vi "Open DQMH MHL Request Case QD.vi"(6 "Variant in":variant, 7 "Shift Pressed?":bool, 8 "error in (no error)":errorcluster, 10 "QD Combo Box Ref":refnum<vi>, 11 "QD Launch VI Ref":refnum<vi>) -> (0 "error out":errorcluster, 4 "Variant out":variant)   [LabVIEW 2017]
doc: "Write a 1-2 sentence description of the functionality of your plugin here. Replace the \"$\" below with the character you wish to assign as the default shortcut for this plugin. Do not add any text after the 'Default Shortcut' line below.\n\nDefault Shortcut - [k]"
panel:
  in  "Undo Name":string="Quick Drop Keyboard Shortcut"
  # "Do not change the connector pane of this VI.\n\nSee the block diagram for directions on how to use this template."
  # "Specify the name of the Undo transaction"
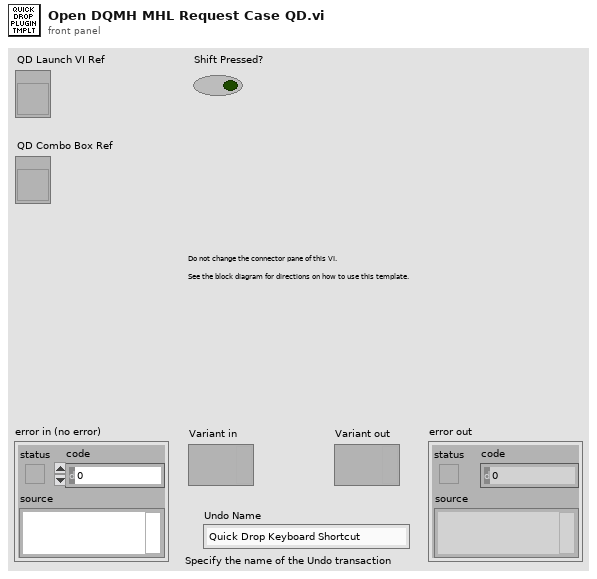
[diagram p1: front panel]
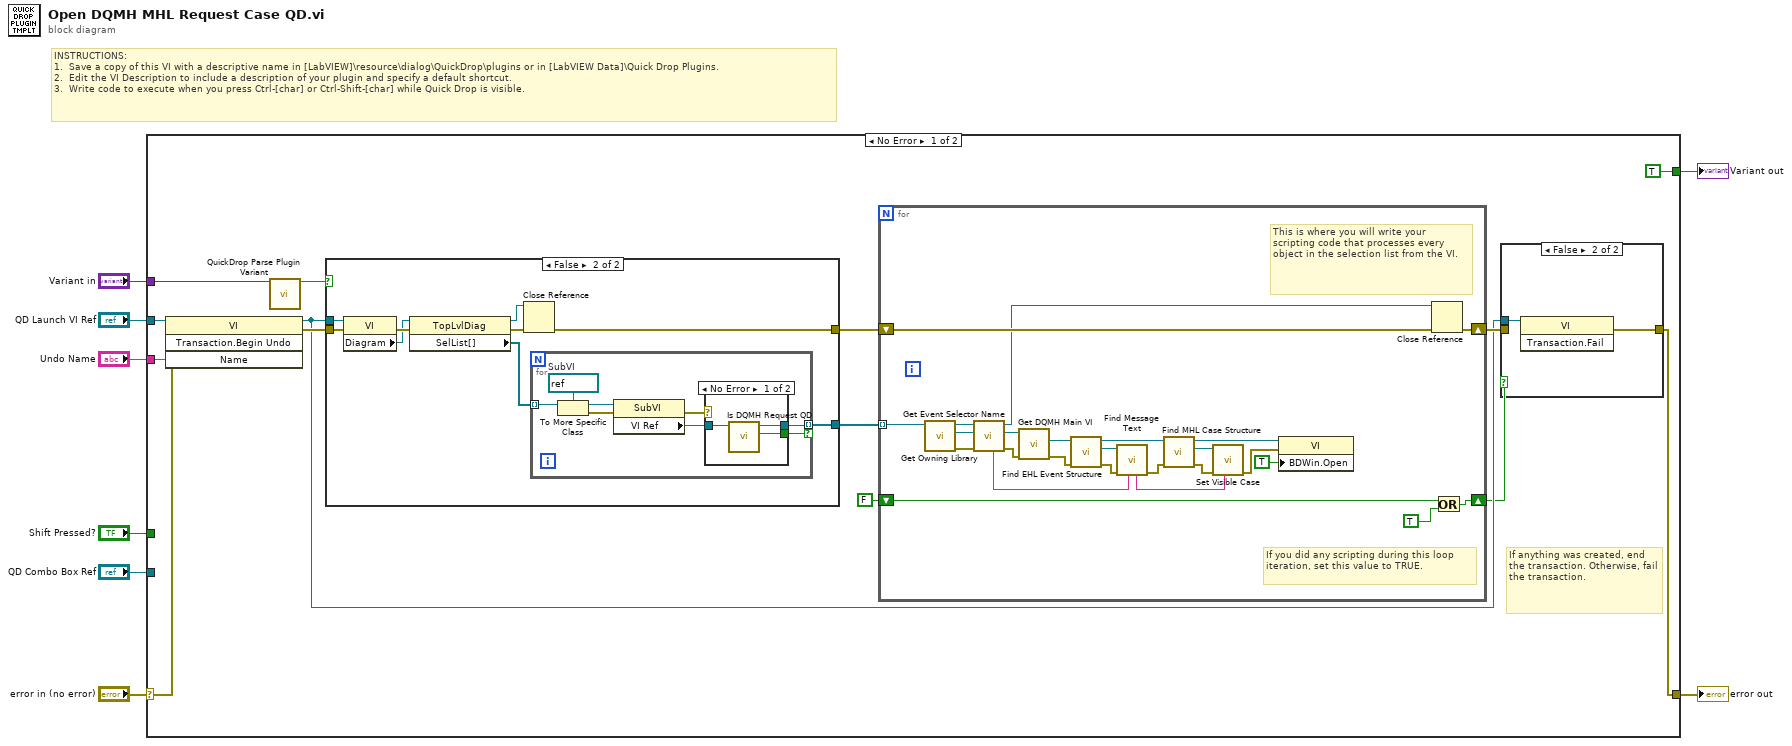
[diagram p0: block diagram]
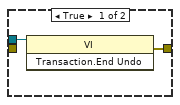
[diagram p2: hidden frame]
diagram:
  # "INSTRUCTIONS:\n1.  Save a copy of this VI with a descriptive name in [LabVIEW]\\resource\\dialog\\QuickDrop\\plugins or in [LabVIEW Data]\\Quick Drop Plugins.\n2.  Edit the VI Description to include a description of your plugin and specify a default shortcut. \n3.  Write code to execute when you press Ctrl-[char] or Ctrl-Shift-[char] while Quick Drop is visible."
  n1 = case shown="No Error" "error in (no error)" {
    selector: "error in (no error)" -> [w21 w73]
    tunnel: [w15 w73] -> w7
    tunnel: "QD Launch VI Ref" -> [w20 _]
    tunnel: "Shift Pressed?" -> [_ _]
    tunnel: "QD Combo Box Ref" -> [_ _]
    tunnel: "Variant in" -> [w22 _]
    tunnel: "Undo Name" -> [w19 _]
    tunnel: [TRUE _] -> w1
    frame No Error {
      # "If anything was created, end the transaction. Otherwise, fail the transaction."
      n2 = invoke class="VI" method="Transaction.Begin Undo"(reference=w20, error in=w21, "Name"=w19) -> (reference out=w12:refnum<vi>, error out=w16:errorcluster)  [unwired: 1 in, 2 out]
      n3 = call <vilib>:"QuickDrop Parse Plugin Variant.vi"("QDKS Variant in"=w22) -> ("QD Launch VI Panel?"=w17:bool)  [unwired: 12 in, 2 out]
      n4 = case shown="False" w17 {
        tunnel: w16 -> [w52 w61]
        tunnel: w12 -> [_ w60]
        tunnel: [w52 w55] -> w14
        tunnel: [_ w53] -> w9
        frame True {
        }
        frame False {
          n5 = property class="VI"(reference=w60, error in=w61) -> (error out=w59:errorcluster, "Diagram"=w58:refnum<vi>)  [unwired: 1 out]
          n6 = property class="TopLvlDiag"(reference=w58, error in=w59) -> (reference out=w56:refnum<vi>, error out=w57:errorcluster, "SelList[]"=w54:refnum<vi>[])
          n7 = Close Reference(reference=w56, error in (no error)=w57) -> (error out=w55:errorcluster)
          n8 = for {
            tunnel: w54 -> [w68] mode=indexing
            tunnel: [w62] -> w53 mode=indexing if=w67
            w69 = refnum<vi> refnum  # SubVI
            n9 = To More Specific Class(target class=w69, reference=w68) -> (specific class reference=w66:refnum<vi>, error out=w65:errorcluster)  [unwired: 1 in]
            n10 = property class="SubVI"(reference=w66, error in=w65) -> (error out=w64:errorcluster, "VI Ref"=w63:refnum<vi>)  [unwired: 1 out]
            n11 = case shown="No Error" w64 {
              tunnel: [w70 _] -> w67
              tunnel: w63 -> [w72 _]
              tunnel: [w71 _] -> w62
              frame No Error {
                n12 = call "Is DQMH Request QD.vi"("VI in"=w72) -> ("Is a DQMH Request"=w70:bool, "VI out"=w71:refnum<vi>)  [unwired: 8 in, 1 out]
              }
              frame Error {
              }
            }
          }
        }
      }
      n13 = for {
        shift-right: [w43] -> w13
        shift-left: w14 -> [w44]
        shift-right: [w46] -> w10
        shift-left: FALSE -> [w47]
        tunnel: w9 -> [w38] mode=indexing
        # "This is where you will write your scripting code that processes every object in the selection list from the VI."
        # "If you did any scripting during this loop iteration, set this value to TRUE."
        n14 = call "Get Owning Library.vi"("VI in"=w38) -> ("error out"=w40:errorcluster, "Owning Library"=w42:refnum<vi>, "VI out"=w41:refnum<vi>)  [unwired: 7 in, 1 out]
        n15 = call "Get Event Selector Name.vi"("error in (no error)"=w40, "Library Ref in"=w42, "VI Ref in"=w41) -> ("error out"=w30:errorcluster, "Library Ref out"=w39:refnum<vi>, "VI Ref out"=w23:refnum<vi>, "Event Selector Name"=w35:string)  [unwired: 5 in]
        n16 = call "Get DQMH Main VI.vi"("error in (no error)"=w30, "Library Ref in"=w39) -> ("error out"=w31:errorcluster, "Main VI Ref"=w37:refnum<vi>)  [unwired: 7 in, 1 out]
        n17 = call "Find EHL Event Structure.vi"("error in (no error)"=w31, "VI Ref in"=w37) -> ("error out"=w32:errorcluster, "EHL Event Structure"=w36:refnum<vi>, "VI Ref out"=w34:refnum<vi>)  [unwired: 6 in, 1 out]
        n18 = call "Find Message Text.vi"("Event Selector Name"=w35, "error in (no error)"=w32, "EventStructure in"=w36) -> ("error out"=w33:errorcluster, "Message Text"=w28:string)  [unwired: 7 in]
        n19 = call "Find MHL Case Structure.vi"("error in (no error)"=w33, "VI Ref in"=w34) -> ("error out"=w26:errorcluster, "MHL Case Structure"=w29:refnum<vi>, "VI Ref out"=w27:refnum<vi>)  [unwired: 6 in, 1 out]
        n20 = call "Set Visible Case.vi"("Message Text"=w28, "error in (no error)"=w26, "CaseStructure in"=w29) -> ("error out"=w25:errorcluster)  [unwired: 8 in]
        n21 = property class="VI"(reference=w27, error in=w25, "BDWin.Open"=TRUE ("Block Diagram Window:Open")) -> ()  [unwired: 2 out]
        n22 = Close Reference(reference=w23, error in (no error)=w44) -> (error out=w43:errorcluster)
        n23 = Or(x=w47, y=TRUE ("x")) -> (x .or. y?=w46:bool)
      }
      n24 = case shown="False" w10 {
        tunnel: w12 -> [w48 w50]
        tunnel: [w49 w51] -> w15
        tunnel: w13 -> [_ _]
        frame True {
          n25 = invoke class="VI" method="Transaction.End Undo"(reference=w48) -> (error out=w49:errorcluster)  [unwired: 2 in, 2 out]
        }
        frame False {
          n26 = invoke class="VI" method="Transaction.Fail"(reference=w50) -> (error out=w51:errorcluster)  [unwired: 2 in, 2 out]
        }
      }
    }
    frame Error {
    }
  }
  "error out" <- w7
  "Variant out" <- w1
